vi "Untitled 5.vi"() -> ()   [LabVIEW 2021]
panel:
  in  "Температура снаружи":dbl
  in  "kd":dbl
  out "XY Graph":cluster{i32[], dbl[]}[](graph)
  in  "stop":bool
  in  "ki":dbl
  in  "kp":dbl
  out "IprevErr":dbl
  in  "dt":dbl
  out "I":dbl
  out "Даткчик":dbl
  in  "Установка":dbl
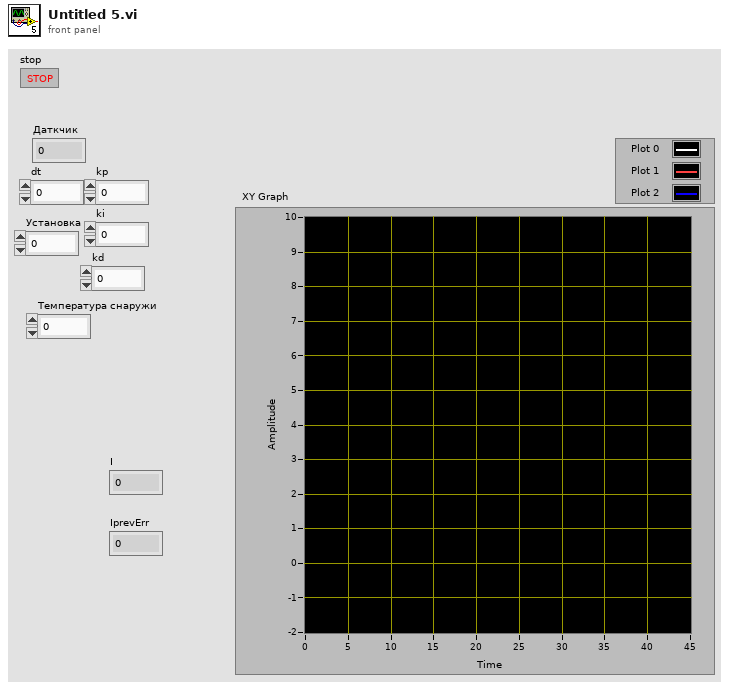
[diagram p1: front panel]
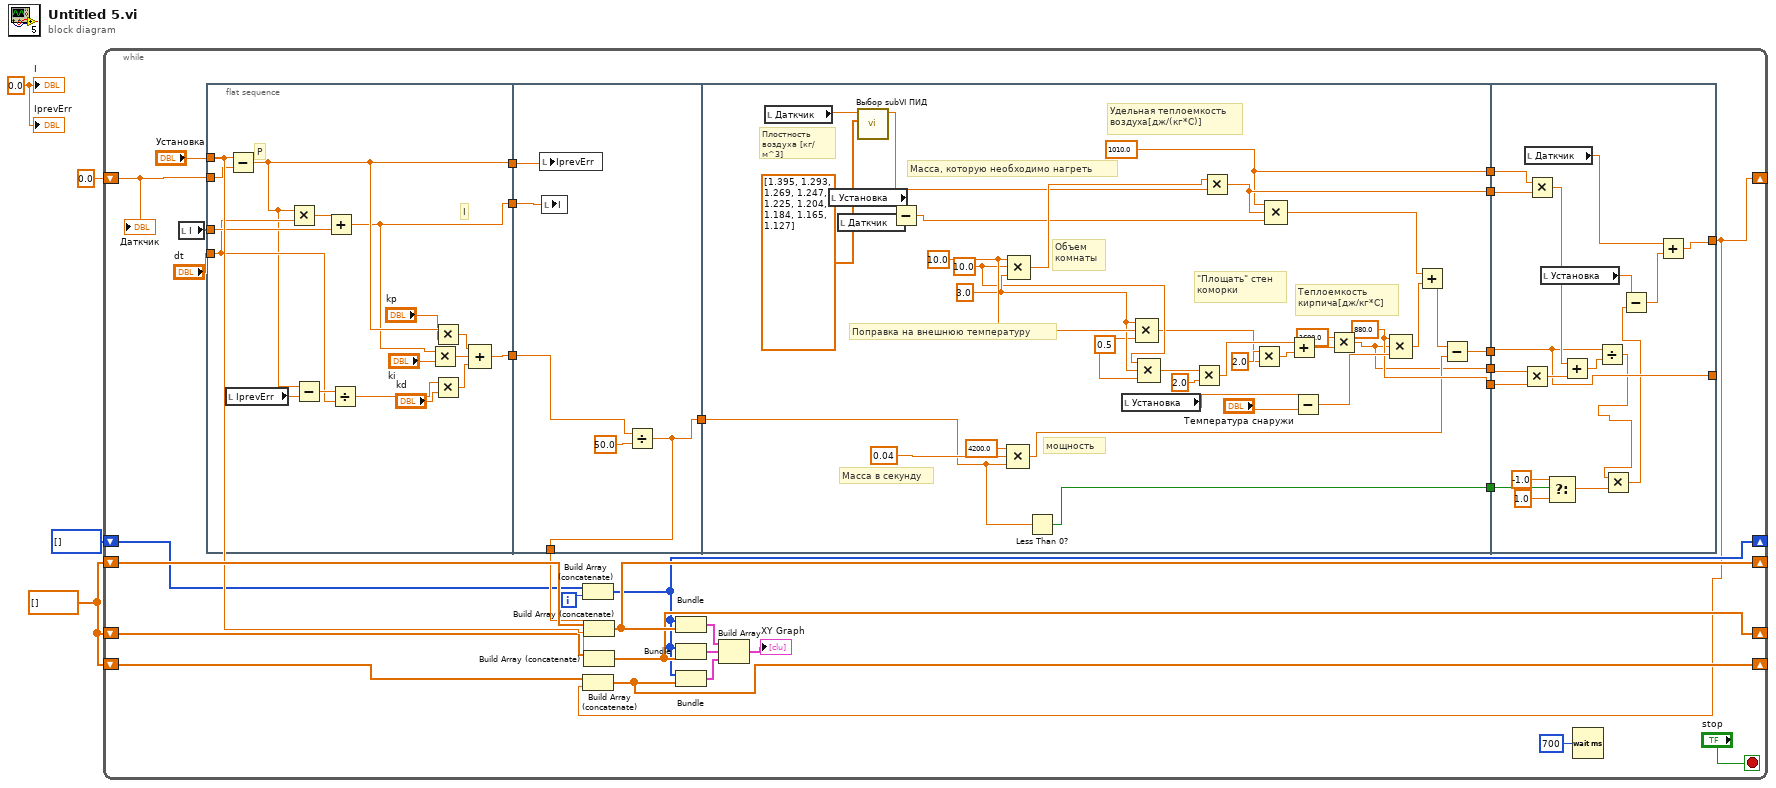
[diagram p0: block diagram]
diagram:
  w1 = 0.0 ("I")
  w3 = dbl[] []
  n1 = while {
    shift-right: [w18] -> _
    shift-left: i32[] [] -> [w20]
    shift-right: [w22] -> _
    shift-left: w3 -> [w28]
    shift-right: [w21] -> _
    shift-left: w3 -> [w26]
    shift-right: [w15] -> _
    shift-left: w3 -> [w17]
    shift-right: [w6] -> _
    shift-left: 0.0 -> [w8]
    i -> [w19]
    stop <- "stop" stop-if-true
    n2 = local read "I"() -> (w34:dbl)
    n3 = flat-sequence {
      tunnel: "Установка" -> [w50]
      tunnel: w8 -> [w49]
      tunnel: "dt" -> [w46]
      tunnel: w34 -> [w51]
      tunnel: [w40] -> w33
      tunnel: [w41] -> w32
      tunnel: [w45] -> w31
      tunnel: w33 -> [w57]
      tunnel: w32 -> [w56]
      tunnel: w31 -> [w54]
      tunnel: [w53] -> w23
      tunnel: [w53] -> w16
      tunnel: w16 -> [w65]
      tunnel: [w74] -> w14
      tunnel: [w73] -> w13
      tunnel: [w58] -> w12
      tunnel: [w72] -> w11
      tunnel: [w71] -> w10
      tunnel: [w64] -> w5
      tunnel: w14 -> [w103]
      tunnel: w13 -> [w109]
      tunnel: w12 -> [w107]
      tunnel: w11 -> [w110]
      tunnel: w10 -> [w108]
      tunnel: [w103] -> _
      tunnel: [w102] -> w6
      tunnel: w5 -> [w99]
      frame #0 {
        # "I"
        # "P"
        n4 = local read "IprevErr"() -> (w48:dbl)
        n5 = Subtract(x=w50, y=w49) -> (x-y=w41:dbl)
        n6 = Multiply(x=w41, y=w46) -> (x*y=w52:dbl)
        n7 = Subtract(x=w41, y=w48) -> (x-y=w47:dbl)
        n8 = Add(x=w52, y=w51) -> (x+y=w40:dbl)
        n9 = Divide(x=w47, y=w46) -> (x/y=w39:dbl)
        n10 = Multiply(x=w40, y="ki") -> (x*y=w43:dbl)
        n11 = Multiply(x=w41, y="kp") -> (x*y=w44:dbl)
        n12 = Multiply(x=w39, y="kd") -> (x*y=w42:dbl)
        n13 = Compound Arithmetic op=ADD(w44, w43, w42) -> (w45:dbl)
      }
      frame #1 {
        n14 = local write "IprevErr"(w56) -> ()
        n15 = local write "I"(w57) -> ()
        n16 = Divide(x=w54, y=50.0) -> (x/y=w53:dbl)
      }
      frame #2 {
        w86 = 0.5 ("value")
        w71 = 880.0 ("value")
        w72 = 1010.0 ("value")
        w82 = 10.0 ("value")
        w87 = 3.0 ("value")
        w88 = 10.0 ("value")
        # "мощность"
        # "Масса в секунду"
        # "\"Площать\" стен\nкоморки"
        # "Теплоемкость\nкирпича[дж/кг*С]"
        # "Поправка на внешнюю температуру"
        # "Удельная теплоемкость\nвоздуха[дж/(кг*С)]"
        # "Масса, которую необходимо нагреть"
        # "Плостность \nвоздуха [кг/м^3]"
        # "Объем \nкомнаты"
        n17 = local read "Даткчик"() -> (w61:dbl)
        n18 = local read "Установка"() -> (w62:dbl)
        n19 = local read "Даткчик"() -> (w80:dbl)
        n20 = call "Выбор subVI ПИД.vi"("Array"=dbl[] [1.395, 1.293, 1.269, 1.247, 1.225, 1.204, 1.184, 1.165, 1.127], "Температура\nдома"=w61) -> ("Numeric"=w78:dbl)  [unwired: 9 in]
        n21 = Subtract(x=w62, y=w80) -> (x-y=w69:dbl)
        n22 = Compound Arithmetic op=MULTIPLY(4200.0 ("value"), 0.04 ("value"), w65) -> (w66:dbl)
        n23 = Compound Arithmetic op=MULTIPLY(w88, w82, w87) -> (w79:dbl)
        n24 = Less Than 0?(x=w65) -> (x < 0?=w64:bool)
        n25 = local read "Установка"() -> (w70:dbl)
        n26 = Compound Arithmetic op=MULTIPLY(w87, w88, w86) -> (w76:dbl)
        n27 = Compound Arithmetic op=MULTIPLY(w82, w87, w86) -> (w83:dbl)
        n28 = Multiply(x=w83, y=2.0) -> (x*y=w89:dbl)
        n29 = Multiply(x=w79, y=w78) -> (x*y=w73:dbl)
        n30 = Multiply(x=2.0 ("y"), y=w76) -> (x*y=w90:dbl)
        n31 = Compound Arithmetic op=MULTIPLY(w72, w73, w69) -> (w91:dbl)
        n32 = Add(x=w89, y=w90) -> (x+y=w60:dbl)
        n33 = Subtract(x=w70, y="Температура снаружи") -> (x-y=w81:dbl)
        n34 = Multiply(x=1600.0, y=w60) -> (x*y=w58:dbl)
        n35 = Compound Arithmetic op=MULTIPLY(w71, w58, w81) -> (w92:dbl)
        n36 = Add(x=w91, y=w92) -> (x+y=w75:dbl)
        n37 = Subtract(x=w75, y=w66) -> (x-y=w74:dbl)
      }
      frame #3 {
        n38 = Multiply(x=w107, y=w108) -> (x*y=w106:dbl)
        n39 = local read "Даткчик"() -> (w101:dbl)
        n40 = Multiply(x=w110, y=w109) -> (x*y=w105:dbl)
        n41 = local read "Установка"() -> (w100:dbl)
        n42 = Select(t=-1.0, s=w99, f=1.0) -> (s? t:f=w98:dbl)
        n43 = Add(x=w105, y=w106) -> (x+y=w104:dbl)
        n44 = Divide(x=w103, y=w104) -> (x/y=w93:dbl)
        n45 = Multiply(x=w93, y=w98) -> (x*y=w95:dbl)
        n46 = Subtract(x=w100, y=w95) -> (x-y=w94:dbl)
        n47 = Add(x=w101, y=w94) -> (x+y=w102:dbl)
      }
    }
    n48 = Build Array (concatenate)(w20, w19) -> (w18:i32[])
    n49 = Build Array (concatenate)(w17, w6) -> (w15:dbl[])
    n50 = Build Array (concatenate)(w28, "Установка") -> (w22:dbl[])
    n51 = Build Array (concatenate)(w26, w23) -> (w21:dbl[])
    n52 = Bundle(w18, w22) -> (w29:cluster{i32[], dbl[]})  [unwired: 1 in]
    n53 = Bundle(w18, w21) -> (w25:cluster{i32[], dbl[]})  [unwired: 1 in]
    n54 = Bundle(w18, w15) -> (w9:cluster{i32[], dbl[]})  [unwired: 1 in]
    n55 = Build Array(w29, w25, w9) -> (→"XY Graph":cluster{i32[], dbl[]}[])
    n56 = Wait (ms)(milliseconds to wait=u32 700) -> ()  [unwired: 1 out]
    "Даткчик" <- w8
  }
  "I" <- w1
  "IprevErr" <- w1
